vi "Pre-Build Action - visa.vi"(6 "Top Level/Always Included VIs":path[](array[path]), 7 "Main Destination Path":path, 9 "Target Name":string, 10 "Build Specification Name":string, 11 "Project Path":path) -> (0 "error out":errorcluster)   [LabVIEW 2013]
doc: "This vi is called by build as pre-build action. VI setup conditional symbols."
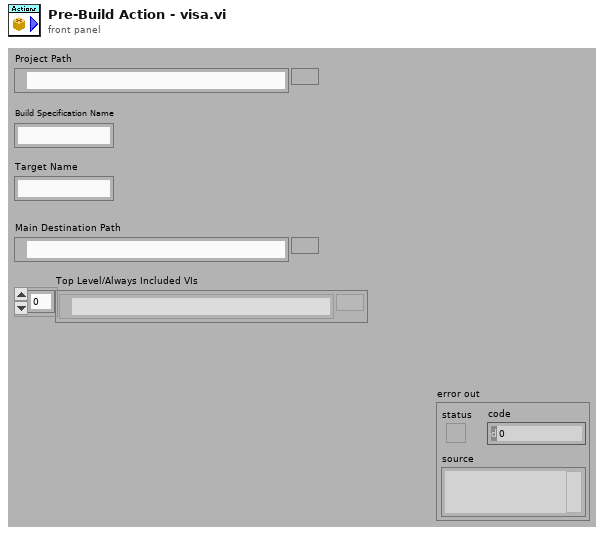
[diagram p1: front panel]
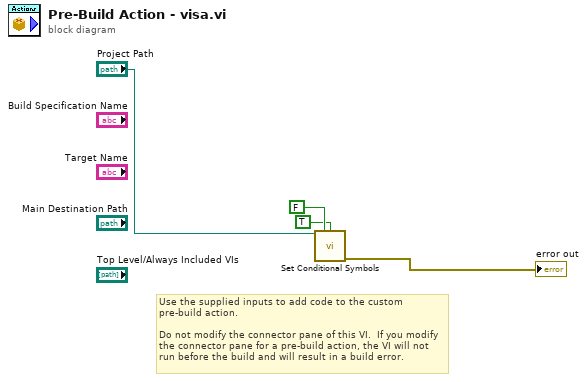
[diagram p0: block diagram]
diagram:
  # "Use the supplied inputs to add code to the custom pre-build action.\n\nDo not modify the connector pane of this VI.  If you modify the connector pane for a pre-build action, the VI will not run before the build and will result in a build error."
  n1 = call "Set Conditional Symbols.vi"("Project Path"="Project Path", "w_niscope"=FALSE, "w_visa"=TRUE) -> ("error out"=→"error out":errorcluster)  [unwired: 12 in]
